vi "to string 2.0.vi"(8 "error in (no error)":errorcluster, 10 "data in":string, 11 "PID Module configuration in":refnum<class "PID Module configuration.lvclass">) -> (0 "error out":errorcluster, 2 "data out":string, 3 "PID Module configuration out":refnum<class "PID Module configuration.lvclass">)   [LabVIEW 2015, in "PID Module configuration.lvclass"]
uses:
  PID Module configuration.lvclass
  PID Module configuration.lvclass/PID Module configuration.ctl
  <vilib>/NI/Tag Bus Module Framework/channel/TBM channel.lvclass
  <vilib>/NI/Configuration Framework/serializable configuration/NISE_CEF_serializable configuration.lvclass
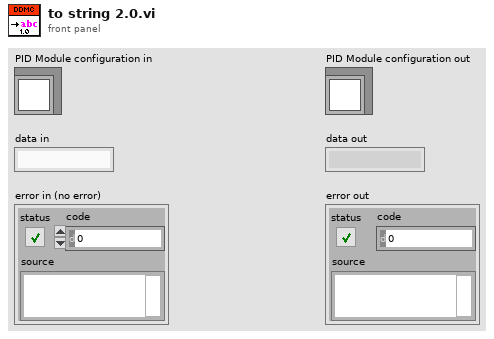
[diagram p1: front panel]
types:
  T1 = typedef "PID Module configuration.lvclass/Line.ctl" = cluster{"PID ID":string, "Setpoint":refnum<class "TBM channel.lvclass">, "Variable":refnum<class "TBM channel.lvclass">, "Output":refnum<class "TBM channel.lvclass">, "Output High":refnum<class "TBM channel.lvclass">, "Output Low":refnum<class "TBM channel.lvclass">, "P":refnum<class "TBM channel.lvclass">, "I":refnum<class "TBM channel.lvclass">, "D":refnum<class "TBM channel.lvclass">}
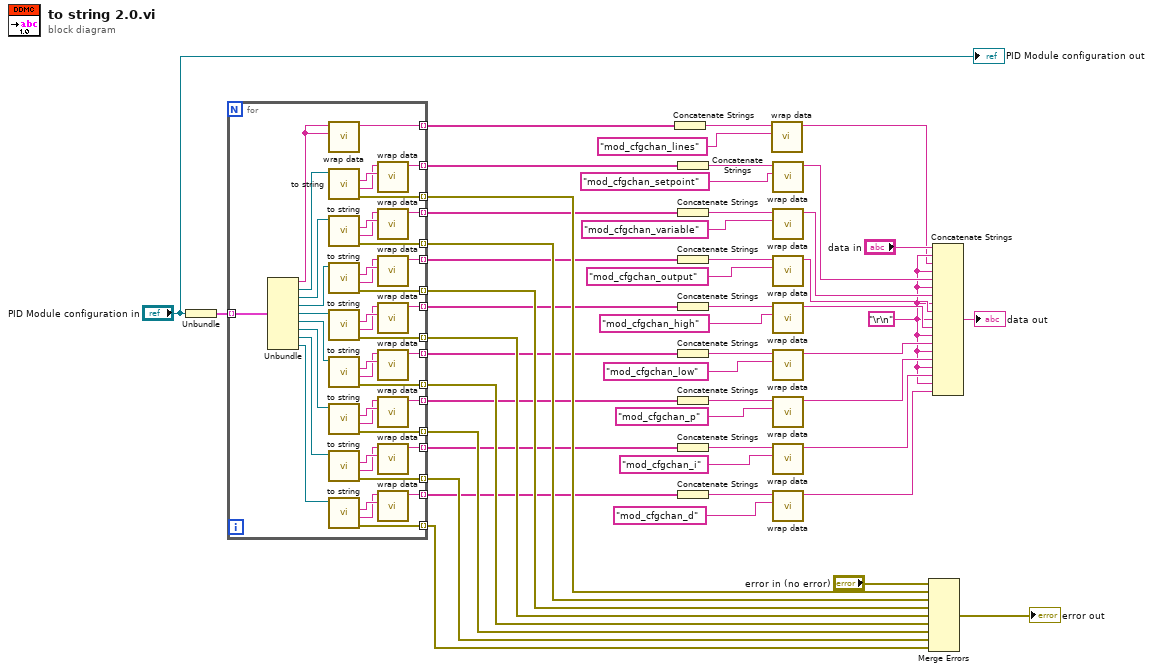
[diagram p0: block diagram]
diagram:
  w10 = "\r\n"
  n1 = Unbundle("PID Module configuration in") -> (w46:T1[])
  n2 = for {
    tunnel: w46 -> [w94] mode=indexing
    tunnel: [w91] -> w47 mode=indexing
    tunnel: [w90] -> w51 mode=indexing
    tunnel: [w88] -> w1 mode=indexing
    tunnel: [w74] -> w42 mode=indexing
    tunnel: [w73] -> w41 mode=indexing
    tunnel: [w72] -> w40 mode=indexing
    tunnel: [w71] -> w39 mode=indexing
    tunnel: [w70] -> w38 mode=indexing
    tunnel: [w69] -> w37 mode=indexing
    tunnel: [w62] -> w30 mode=indexing
    tunnel: [w61] -> w29 mode=indexing
    tunnel: [w60] -> w28 mode=indexing
    tunnel: [w59] -> w27 mode=indexing
    tunnel: [w58] -> w26 mode=indexing
    tunnel: [w57] -> w25 mode=indexing
    tunnel: [w53] -> w20 mode=indexing
    tunnel: [w52] -> w18 mode=indexing
    n3 = Unbundle(w94) -> ("PID ID"=w89:string, "Setpoint"=w87:refnum<class "TBM channel.lvclass">, "Variable"=w80:refnum<class "TBM channel.lvclass">, "Output"=w79:refnum<class "TBM channel.lvclass">, "Output High"=w78:refnum<class "TBM channel.lvclass">, "Output Low"=w77:refnum<class "TBM channel.lvclass">, "P"=w76:refnum<class "TBM channel.lvclass">, "I"=w75:refnum<class "TBM channel.lvclass">, "D"=w56:refnum<class "TBM channel.lvclass">)
    n4 = call <vilib>:"wrap data.vi"("identifier"=w89, "data to wrap"=w89) -> ("wrapped data"=w88:string)  [unwired: 9 in]
    n5 = call-dynamic "to string.vi"("channel in"=w87) -> ("error out"=w90:errorcluster, "channel data"=w92:string, "identifier"=w93:string)  [unwired: 7 in, 1 out]
    n6 = call-dynamic "to string.vi"("channel in"=w80) -> ("error out"=w74:errorcluster, "channel data"=w68:string, "identifier"=w86:string)  [unwired: 7 in, 1 out]
    n7 = call-dynamic "to string.vi"("channel in"=w79) -> ("error out"=w73:errorcluster, "channel data"=w67:string, "identifier"=w85:string)  [unwired: 7 in, 1 out]
    n8 = call-dynamic "to string.vi"("channel in"=w78) -> ("error out"=w72:errorcluster, "channel data"=w66:string, "identifier"=w84:string)  [unwired: 7 in, 1 out]
    n9 = call-dynamic "to string.vi"("channel in"=w77) -> ("error out"=w71:errorcluster, "channel data"=w65:string, "identifier"=w83:string)  [unwired: 7 in, 1 out]
    n10 = call-dynamic "to string.vi"("channel in"=w76) -> ("error out"=w70:errorcluster, "channel data"=w64:string, "identifier"=w82:string)  [unwired: 7 in, 1 out]
    n11 = call-dynamic "to string.vi"("channel in"=w75) -> ("error out"=w69:errorcluster, "channel data"=w63:string, "identifier"=w81:string)  [unwired: 7 in, 1 out]
    n12 = call-dynamic "to string.vi"("channel in"=w56) -> ("error out"=w52:errorcluster, "channel data"=w54:string, "identifier"=w55:string)  [unwired: 7 in, 1 out]
    n13 = call <vilib>:"wrap data.vi"("identifier"=w93, "data to wrap"=w92) -> ("wrapped data"=w91:string)  [unwired: 9 in]
    n14 = call <vilib>:"wrap data.vi"("identifier"=w86, "data to wrap"=w68) -> ("wrapped data"=w62:string)  [unwired: 9 in]
    n15 = call <vilib>:"wrap data.vi"("identifier"=w85, "data to wrap"=w67) -> ("wrapped data"=w61:string)  [unwired: 9 in]
    n16 = call <vilib>:"wrap data.vi"("identifier"=w84, "data to wrap"=w66) -> ("wrapped data"=w60:string)  [unwired: 9 in]
    n17 = call <vilib>:"wrap data.vi"("identifier"=w83, "data to wrap"=w65) -> ("wrapped data"=w59:string)  [unwired: 9 in]
    n18 = call <vilib>:"wrap data.vi"("identifier"=w82, "data to wrap"=w64) -> ("wrapped data"=w58:string)  [unwired: 9 in]
    n19 = call <vilib>:"wrap data.vi"("identifier"=w81, "data to wrap"=w63) -> ("wrapped data"=w57:string)  [unwired: 9 in]
    n20 = call <vilib>:"wrap data.vi"("identifier"=w55, "data to wrap"=w54) -> ("wrapped data"=w53:string)  [unwired: 9 in]
  }
  n21 = Concatenate Strings(w1) -> (w8:string)
  n22 = Concatenate Strings(w47) -> (w48:string)
  n23 = Concatenate Strings(w30) -> (w36:string)
  n24 = Concatenate Strings(w29) -> (w35:string)
  n25 = Concatenate Strings(w28) -> (w34:string)
  n26 = Concatenate Strings(w27) -> (w33:string)
  n27 = Concatenate Strings(w26) -> (w32:string)
  n28 = Concatenate Strings(w25) -> (w31:string)
  n29 = Concatenate Strings(w20) -> (w21:string)
  n30 = call <vilib>:"wrap data.vi"("identifier"="mod_cfgchan_lines", "data to wrap"=w8) -> ("wrapped data"=w2:string)  [unwired: 9 in]
  n31 = call <vilib>:"wrap data.vi"("identifier"="mod_cfgchan_setpoint", "data to wrap"=w48) -> ("wrapped data"=w49:string)  [unwired: 9 in]
  n32 = call <vilib>:"wrap data.vi"("identifier"="mod_cfgchan_variable", "data to wrap"=w36) -> ("wrapped data"=w17:string)  [unwired: 9 in]
  n33 = call <vilib>:"wrap data.vi"("identifier"="mod_cfgchan_output", "data to wrap"=w35) -> ("wrapped data"=w16:string)  [unwired: 9 in]
  n34 = call <vilib>:"wrap data.vi"("identifier"="mod_cfgchan_high", "data to wrap"=w34) -> ("wrapped data"=w15:string)  [unwired: 9 in]
  n35 = call <vilib>:"wrap data.vi"("identifier"="mod_cfgchan_low", "data to wrap"=w33) -> ("wrapped data"=w14:string)  [unwired: 9 in]
  n36 = call <vilib>:"wrap data.vi"("identifier"="mod_cfgchan_p", "data to wrap"=w32) -> ("wrapped data"=w13:string)  [unwired: 9 in]
  n37 = call <vilib>:"wrap data.vi"("identifier"="mod_cfgchan_i", "data to wrap"=w31) -> ("wrapped data"=w12:string)  [unwired: 9 in]
  n38 = call <vilib>:"wrap data.vi"("identifier"="mod_cfgchan_d", "data to wrap"=w21) -> ("wrapped data"=w11:string)  [unwired: 9 in]
  n39 = Merge Errors("error in (no error)", w51, w42, w41, w40, w39, w38, w37, w18) -> (→"error out":errorcluster)
  n40 = Concatenate Strings("data in", w10, w2, w10, w49, w10, w17, w10, w16, w10, w15, w10, w14, w10, w13, w10, w12, w10, w11) -> (→"data out":string)
  "PID Module configuration out" <- "PID Module configuration in"
